vi "456.vi"(1 "逆运动学输入":dbl[](array[numeric])=[0.2, 0.0, 0.3], 2 "123":dbl[](array[numeric]), 3 "机械臂末端姿态":dbl[][](array[numeric])) -> (0 "逆运动学输出":dbl[](array[numeric])=[0.0, 90.0, 0.0, 0.0, -90.0, -0.0] format="%#.3f")   [LabVIEW 2015]
uses:
  <vilib>/Utility/file.llb/Read From Spreadsheet File (DBL).vi
panel:
  out "angle42":dbl
  out "3角度输出":dbl[](array[numeric])
  out "角度/弧度":dbl
  out "弧度/角度":dbl
  out "az":dbl=1.0
  out "ay":dbl
  out "ax":dbl
  out "angle6":dbl
  out "angle5":dbl
  out "angle4":dbl
  out "angle3":dbl
  out "angle2":dbl
  out "angle1":dbl
  in  "机械臂臂长":dbl[](array[numeric])=[558.0, 764.0, 993.0, 420.0]
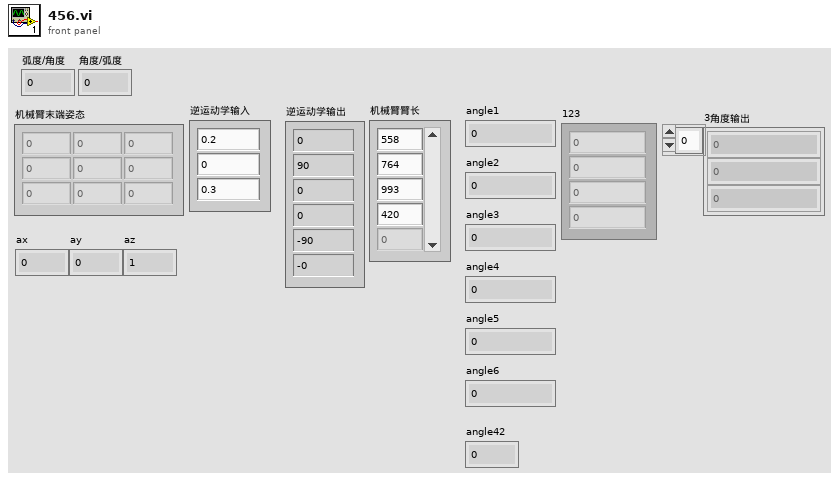
[diagram p1: front panel]
types:
  T1 = typedef "Real Matrix NI_Silver.ctl" = dbl[][]
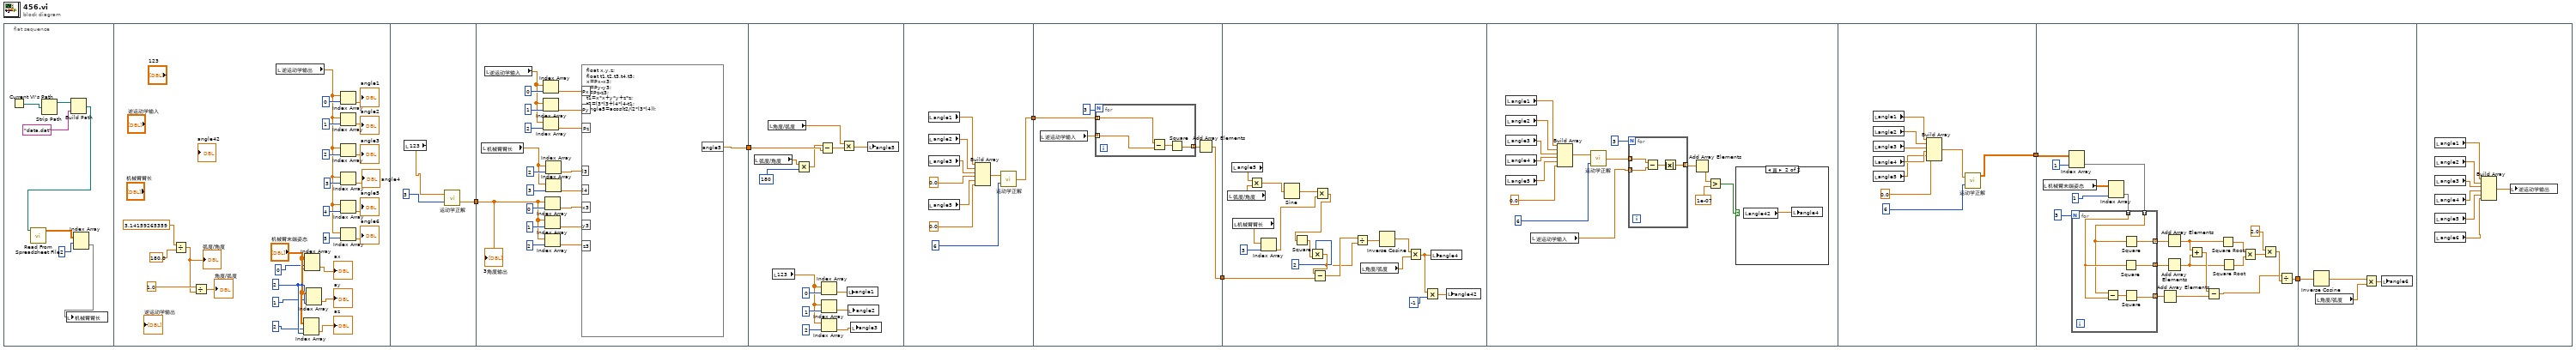
[diagram p0: block diagram]
diagram:
  n1 = flat-sequence {
    tunnel: [w41] -> w2
    tunnel: [w43] -> w6
    tunnel: w2 -> [w55]
    tunnel: w6 -> [w64]
    tunnel: [w78] -> w5
    tunnel: w5 -> [w88]
    tunnel: [w86] -> w4
    tunnel: w4 -> [w111]
    tunnel: [w134] -> w1
    tunnel: w1 -> [w162]
    tunnel: [w143] -> w3
    tunnel: w3 -> [w173]
    frame #0 {
      n2 = Current VI's Path() -> (path=w10:path)
      n3 = Strip Path(path=w10) -> (stripped path=w9:path)  [unwired: 1 out]
      n4 = Build Path(base path=w9, name or relative path="data.dat") -> (appended path=w7:path)
      n5 = call-poly <vilib>:"Read From Spreadsheet File.vi"("file path (dialog if empty)"=w7) -> ("all rows"=w13:dbl[][])  [unwired: 6 in, 4 out]
      n6 = Index Array(array=w13, index (row)=2) -> (element=w12:dbl[])  [unwired: 1 in]
      n7 = local write "机械臂臂长"(w12) -> ()
    }
    frame #1 {
      w23 = 2
      n8 = Divide(x=3.14159265359, y=180.0) -> (x/y=w15:dbl)
      "弧度/角度" <- w15
      n9 = Divide(x=1.0, y=w15) -> (x/y=→"角度/弧度":dbl)
      n10 = local read "逆运动学输出"() -> (w27:dbl[])
      n11 = Index Array(array="机械臂末端姿态", index (row)=2, index (col)=w23) -> (element=→"az":dbl)
      n12 = Index Array(array="机械臂末端姿态", index (row)=0, index (col)=w23) -> (element=→"ax":dbl)
      n13 = Index Array(array="机械臂末端姿态", index (row)=1, index (col)=w23) -> (element=→"ay":dbl)
      n14 = Index Array(array=w27, index=0) -> (element=→"angle1":dbl)
      n15 = Index Array(array=w27, index=1) -> (element=→"angle2":dbl)
      n16 = Index Array(array=w27, index=2) -> (element=→"angle3":dbl)
      n17 = Index Array(array=w27, index=3) -> (element=→"angle4":dbl)
      n18 = Index Array(array=w27, index=4) -> (element=→"angle5":dbl)
      n19 = Index Array(array=w27, index=5) -> (element=→"angle6":dbl)
    }
    frame #2 {
      n20 = local read "123"() -> (w40:dbl[])
      n21 = call "运动学正解.vi"("正运动学输入"=w40, "关节数"=3) -> ("腕部输出"=w41:dbl[])  [unwired: 2 out]
    }
    frame #3 {
      n22 = local read "机械臂臂长"() -> (w46:dbl[])
      n23 = local read "逆运动学输入"() -> (w59:dbl[])
      n24 = Index Array(array=w59, index=0) -> (element=w49:dbl)
      n25 = Index Array(array=w59, index=1) -> (element=w50:dbl)
      n26 = Index Array(array=w59, index=2) -> (element=w51:dbl)
      n27 = Index Array(array=w55, index=0) -> (element=w54:dbl)
      n28 = Index Array(array=w55, index=1) -> (element=w53:dbl)
      n29 = Index Array(array=w55, index=2) -> (element=w52:dbl)
      n30 = Index Array(array=w46, index=2) -> (element=w45:dbl)
      n31 = Index Array(array=w46, index=3) -> (element=w44:dbl)
      n32 = formula code="float x,y,z;\nfloat t1,t2,t3,t4,t5;\nx=Px-x3;\ny=Py-y3;\nz=Pz-z3;\nt1=x*x+y*y+z*z;\nt2=l3*l3+l4*l4-t1;\nangle5=acos(t2/(2*l3*l4));"("Px"=w49, "Py"=w50, "Pz"=w51, "x3"=w54, "y3"=w53, "z3"=w52, "l4"=w44, "l3"=w45) -> ("angle5"=w43:dbl)
      "3角度输出" <- w55
    }
    frame #4 {
      n33 = local read "弧度/角度"() -> (w76:dbl)
      n34 = local read "角度/弧度"() -> (w66:dbl)
      n35 = local read "123"() -> (w71:dbl[])
      n36 = Multiply(x=w76, y=180) -> (x*y=w63:dbl)
      n37 = Subtract(x=w63, y=w64) -> (x-y=w67:dbl)
      n38 = Index Array(array=w71, index=0) -> (element=w70:dbl)
      n39 = Index Array(array=w71, index=1) -> (element=w68:dbl)
      n40 = Index Array(array=w71, index=2) -> (element=w69:dbl)
      n41 = Multiply(x=w66, y=w67) -> (x*y=w65:dbl)
      n42 = local write "angle1"(w70) -> ()
      n43 = local write "angle2"(w68) -> ()
      n44 = local write "angle3"(w69) -> ()
      n45 = local write "angle5"(w65) -> ()
    }
    frame #5 {
      n46 = local read "angle1"() -> (w85:dbl)
      n47 = local read "angle2"() -> (w84:dbl)
      n48 = local read "angle3"() -> (w83:dbl)
      n49 = local read "angle5"() -> (w82:dbl)
      n50 = Build Array(w85, w84, w83, 0.0, w82, 0.0) -> (w79:dbl[])
      n51 = call "运动学正解.vi"("正运动学输入"=w79, "关节数"=6) -> ("正解输出"=w78:dbl[])  [unwired: 2 out]
    }
    frame #6 {
      n52 = local read "逆运动学输入"() -> (w87:dbl[])
      n53 = for {
        N: 3 -> [_]
        tunnel: [w93] -> w89 mode=indexing
        tunnel: w88 -> [w92] mode=indexing
        tunnel: w87 -> [w91] mode=indexing
        n54 = Subtract(x=w92, y=w91) -> (x-y=w94:dbl)
        n55 = Square(x=w94) -> (x^2=w93:dbl)
      }
      n56 = Add Array Elements(numeric array=w89) -> (sum=w86:dbl)
    }
    frame #7 {
      n57 = local read "弧度/角度"() -> (w105:dbl)
      n58 = local read "angle5"() -> (w106:dbl)
      n59 = local read "机械臂臂长"() -> (w113:dbl[])
      n60 = Multiply(x=w106, y=w105) -> (x*y=w104:dbl)
      n61 = Index Array(array=w113, index=3) -> (element=w109:dbl)
      n62 = Sine(x=w104) -> (sin(x)=w110:dbl)
      n63 = Multiply(x=w110, y=w109) -> (x*y=w101:dbl)
      n64 = Square(x=w101) -> (x^2=w100:dbl)
      n65 = Multiply(x=2, y=w100) -> (x*y=w98:dbl)
      n66 = Subtract(x=w98, y=w111) -> (x-y=w108:dbl)
      n67 = Divide(x=w108, y=w98) -> (x/y=w107:dbl)
      n68 = local read "角度/弧度"() -> (w103:dbl)
      n69 = Inverse Cosine(1:w107) -> (0:w102:dbl)
      n70 = Multiply(x=w102, y=w103) -> (x*y=w96:dbl)
      n71 = Multiply(x=w96, y=-1) -> (x*y=w95:dbl)
      n72 = local write "angle4"(w96) -> ()
      n73 = local write "angle42"(w95) -> ()
    }
    frame #8 {
      n74 = local read "angle1"() -> (w128:dbl)
      n75 = local read "angle2"() -> (w127:dbl)
      n76 = local read "angle3"() -> (w126:dbl)
      n77 = local read "angle4"() -> (w125:dbl)
      n78 = local read "angle5"() -> (w124:dbl)
      n79 = local read "逆运动学输入"() -> (w118:dbl[])
      n80 = Build Array(w128, w127, w126, w125, w124, 0.0) -> (w122:dbl[])
      n81 = call "运动学正解.vi"("正运动学输入"=w122, "关节数"=6) -> ("正解输出"=w119:dbl[])  [unwired: 2 out]
      n82 = for {
        N: 3 -> [_]
        tunnel: w119 -> [w133] mode=indexing
        tunnel: w118 -> [w132] mode=indexing
        tunnel: [w130] -> w117 mode=indexing
        n83 = Subtract(x=w133, y=w132) -> (x-y=w131:dbl)
        n84 = Absolute Value(x=w131) -> (abs(x)=w130:dbl)
      }
      n85 = Add Array Elements(numeric array=w117) -> (sum=w116:dbl)
      n86 = Greater?(x=w116, y=1e-07) -> (0:w114:bool)
      n87 = case shown="真" w114 {
        frame False {
        }
        frame True {
          n88 = local read "angle42"() -> (w129:dbl)
          n89 = local write "angle4"(w129) -> ()
        }
      }
    }
    frame #9 {
      n90 = local read "angle1"() -> (w142:dbl)
      n91 = local read "angle2"() -> (w141:dbl)
      n92 = local read "angle3"() -> (w140:dbl)
      n93 = local read "angle4"() -> (w139:dbl)
      n94 = local read "angle5"() -> (w138:dbl)
      n95 = Build Array(w142, w141, w140, w139, w138, 0.0) -> (w136:dbl[])
      n96 = call "运动学正解.vi"("正运动学输入"=w136, "关节数"=6) -> ("Tx"=w134:T1)  [unwired: 2 out]
    }
    frame #10 {
      n97 = local read "机械臂末端姿态"() -> (w160:dbl[][])
      n98 = Index Array(array=w162, index (col)=1) -> (element=w158:dbl[])  [unwired: 1 in]
      n99 = Index Array(array=w160, index (col)=1) -> (element=w157:dbl[])  [unwired: 1 in]
      n100 = for {
        N: 3 -> [_]
        tunnel: w158 -> [w166] mode=indexing
        tunnel: w157 -> [w167] mode=indexing
        tunnel: [w168] -> w156 mode=indexing
        tunnel: [w165] -> w155 mode=indexing
        tunnel: [w164] -> w154 mode=indexing
        n101 = Subtract(x=w166, y=w167) -> (x-y=w169:dbl)
        n102 = Square(x=w167) -> (x^2=w164:dbl)
        n103 = Square(x=w166) -> (x^2=w165:dbl)
        n104 = Square(x=w169) -> (x^2=w168:dbl)
      }
      n105 = Add Array Elements(numeric array=w156) -> (sum=w152:dbl)
      n106 = Add Array Elements(numeric array=w155) -> (sum=w151:dbl)
      n107 = Add Array Elements(numeric array=w154) -> (sum=w150:dbl)
      n108 = Add(x=w151, y=w150) -> (x+y=w153:dbl)
      n109 = Subtract(x=w153, y=w152) -> (x-y=w144:dbl)
      n110 = Square Root(x=w151) -> (sqrt(x)=w148:dbl)
      n111 = Square Root(x=w150) -> (sqrt(x)=w149:dbl)
      n112 = Multiply(x=w148, y=w149) -> (x*y=w147:dbl)
      n113 = Multiply(x=2.0, y=w147) -> (x*y=w145:dbl)
      n114 = Divide(x=w144, y=w145) -> (x/y=w143:dbl)
    }
    frame #11 {
      n115 = Inverse Cosine(1:w173) -> (0:w171:dbl)
      n116 = local read "角度/弧度"() -> (w172:dbl)
      n117 = Multiply(x=w171, y=w172) -> (x*y=w170:dbl)
      n118 = local write "angle6"(w170) -> ()
    }
    frame #12 {
      n119 = local read "angle1"() -> (w180:dbl)
      n120 = local read "angle2"() -> (w179:dbl)
      n121 = local read "angle3"() -> (w178:dbl)
      n122 = local read "angle4"() -> (w177:dbl)
      n123 = local read "angle5"() -> (w176:dbl)
      n124 = local read "angle6"() -> (w175:dbl)
      n125 = Build Array(w180, w179, w178, w177, w176, w175) -> (w174:dbl[])
      n126 = local write "逆运动学输出"(w174) -> ()
    }
  }
